vi "To DVR.vi"(11 "INode":refnum<class "INode.lvclass">) -> (3 "DVR":refnum<data-value>)   [LabVIEW 2023, in "d20.lvlib" / "INode.lvclass"]
uses:
  INode.lvclass
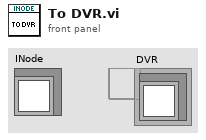
[diagram p1: front panel]
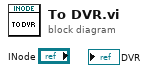
[diagram p0: block diagram]
diagram:
